vi "PID Timing Estimation.vi"(1 "R":bool, 2 "dt (s) in":dbl) -> (7 "dt (s) out":dbl)   [LabVIEW 2019, in "control.lvlib"]
uses:
  control.lvlib
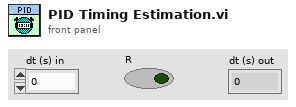
[diagram p1: front panel]
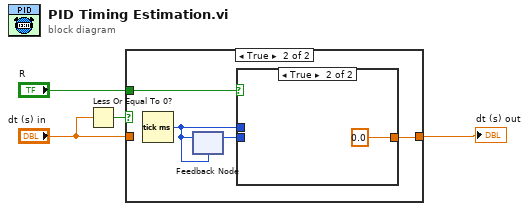
[diagram p0: block diagram]
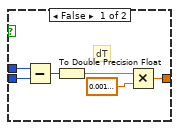
[diagram p3: hidden frame]
diagram:
  n1 = Less Or Equal To 0?(x="dt (s) in") -> (x <= 0?=w1:bool)
  n2 = case shown="True" w1 {
    tunnel: [w5 w6] -> w3
    tunnel: "dt (s) in" -> [w5 _]
    tunnel: "R" -> [_ w9]
    frame False {
    }
    frame True {
      n3 = Tick Count (ms)() -> (millisecond timer value=w7:u32)
      n4 = feedback #1(w7) -> (w8:u32)
      n5 = feedback-in #1(w7) -> ()
      n6 = case shown="True" w9 {
        tunnel: [w10 0.0] -> w6
        tunnel: w8 -> [w14 _]
        tunnel: w7 -> [w15 _]
        frame False {
          # "dT"
          n7 = Subtract(x=w15, y=w14) -> (x-y=w11:u32)
          n8 = To Double Precision Float(number=w11) -> (double precision float=w12:dbl)
          n9 = Multiply(x=w12, y=0.0010000000474974513) -> (x*y=w10:dbl)
        }
        frame True {
        }
      }
    }
  }
  "dt (s) out" <- w3
